vi "Stop Core.vi"(10 "final error code":i32, 11 "Nested in":refnum<class "Camera Worker.lvclass">) -> (3 "Nested out":refnum<class "Camera Worker.lvclass">)   [LabVIEW 2024, in "Camera Worker.lvlib" / "Camera Worker.lvclass"]
doc: "(<B>Filename</B>: Actor Framework.lvlib:Actor.lvclass:Stop Core.vi)\n\nDefines what the actor does before it stops. Use the <B>final error code</B> input to determine whether the actor shut down in response to an error.\n\nBy default, this method does nothing. A descendant class may override it to define behavior, such as shutting down any processes the actor initiated in its override of the Actor Core method."
uses:
  Camera Worker.lvclass
  Camera Worker.lvclass/Camera Worker.ctl
  <vilib>/ActorFramework/Actor/Actor.lvclass
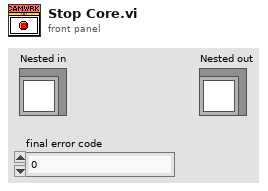
[diagram p1: front panel]
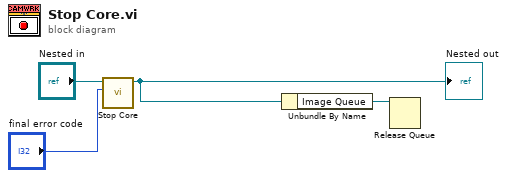
[diagram p0: block diagram]
diagram:
  n1 = call-parent "Stop Core.vi"("final error code"="final error code", "Actor in"="Nested in") -> ("Actor out"=w2:refnum<class "Camera Worker.lvclass">)  [unwired: 9 in]
  "Nested out" <- w2
  n2 = Unbundle By Name(w2) -> ("Image Queue"=w1:refnum<queue>)
  n3 = Release Queue(queue=w1) -> ()  [unwired: 2 in, 3 out]
